vi "Send Pre-Addressed Publish.vi"(8 "error in (no error)":errorcluster, 10 "PublishRequest":refnum<class "PublishRequest.lvclass">, 11 "Publish Message":refnum<class "Publish Msg.lvclass">) -> (0 "error out":errorcluster)   [LabVIEW 2018, in "MVA Framework.lvlib" / "IMediator.lvlib" / "Publish Msg.lvclass"]
doc: "发送发布消息"
uses:
  Publish Msg.lvclass
  composed-af-messages/Source/RoundTripMessage/RoundTripMessage.lvclass
  PublishRequest/PublishRequest.lvclass
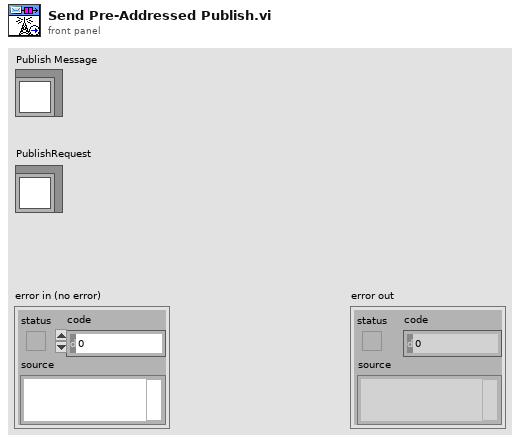
[diagram p1: front panel]
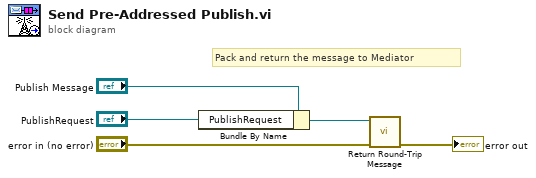
[diagram p0: block diagram]
diagram:
  # "Pack and return the message to Mediator"
  n1 = Bundle By Name(cluster="Publish Message", "PublishRequest"="PublishRequest") -> (w4:refnum<class "Publish Msg.lvclass">)
  n2 = call "Return Round-Trip Message.vi"("error in (no error)"="error in (no error)", "RoundTripMessage In"=w4) -> ("error out"=→"error out":errorcluster)  [unwired: 9 in]
